vi "Write Selected TDMS File.vi"(8 "error in (no error)":errorcluster, 10 "Selected TDMS File":path=path "" caption="start path", 11 "TDMS Data Source in":refnum<class "TDMS Data Source.lvclass">) -> (0 "error out":errorcluster, 3 "TDMS Data Source out":refnum<class "TDMS Data Source.lvclass">)   [LabVIEW 2020, in "TDMS Data Source.lvlib" / "TDMS Data Source.lvclass"]
uses:
  TDMS Data Source.lvclass
  TDMS Data Source.lvclass/TDMS Data Source.ctl
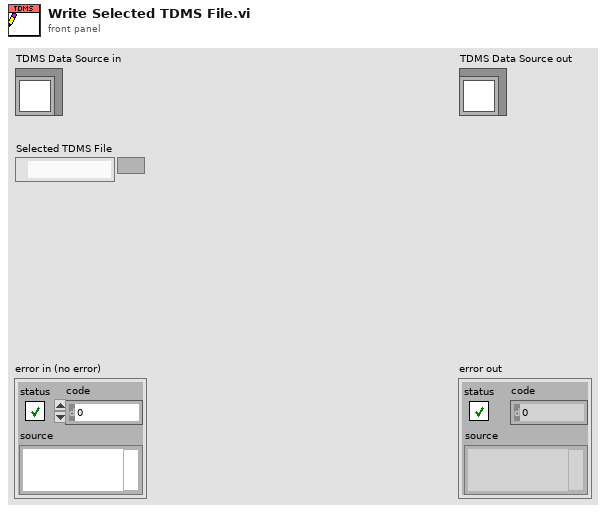
[diagram p1: front panel]
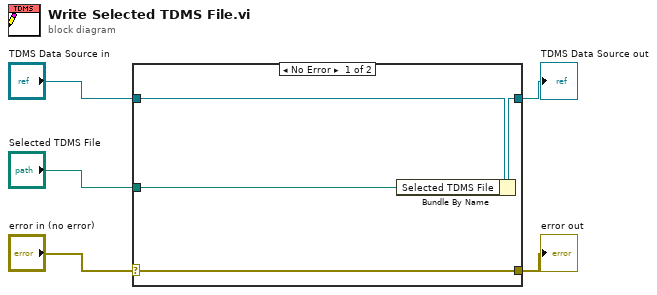
[diagram p0: block diagram]
diagram:
  n1 = case shown="No Error" "error in (no error)" {
    selector: "error in (no error)" -> [w9 w10]
    tunnel: [w9 w10] -> w4
    tunnel: [w7 w11] -> w2
    tunnel: "TDMS Data Source in" -> [w8 w11]
    tunnel: "Selected TDMS File" -> [w6 _]
    frame No Error {
      n2 = Bundle By Name(cluster=w8, "Selected TDMS File"=w6) -> (w7:refnum<class "TDMS Data Source.lvclass">)
    }
    frame Error {
    }
  }
  "error out" <- w4
  "TDMS Data Source out" <- w2
